vi "AttrMap-Merge.vi"(6 "If exist? Skip(T)/Overwrite(F)":bool=TRUE, 8 "error in (no error)":errorcluster, 10 "AttrMap B":T1, 11 "AttrMap A":T1) -> (0 "error out":errorcluster, 3 "AttrMap A after B->A":T1)   [LabVIEW 2019, in "lv-apt-json-file.lvlib"]
uses:
  lv-apt-json-file.lvlib
  Typedef/Def-AttrMap.ctl
  f16f814e-f0a0-47f4-ae2a-f78fd01390a2.vi
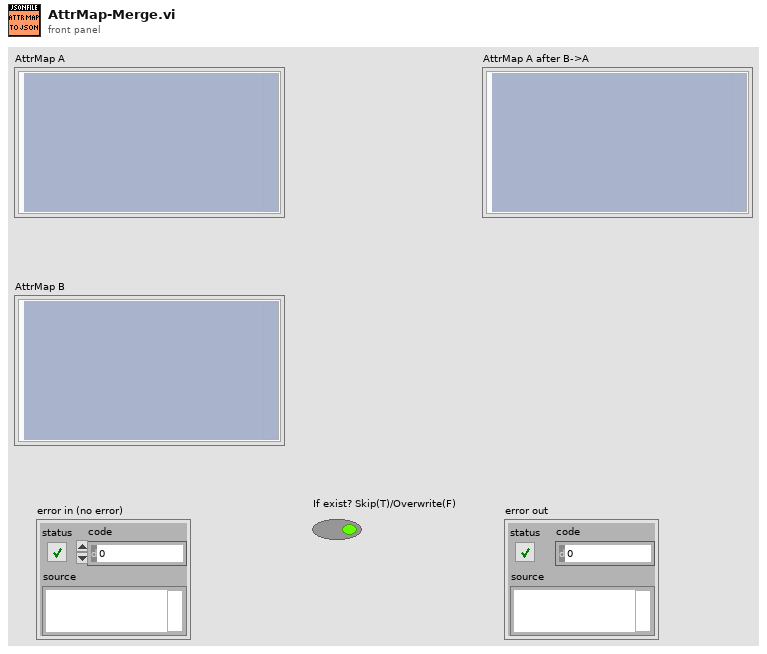
[diagram p1: front panel]
types:
  T1 = typedef "lv-apt-json-file.lvlib/Def-AttrMap.ctl" = cluster{"Map":variant}
  T2 = typedef "lv-apt-json-file.lvlib/Def-NameMap.ctl" = variant[]
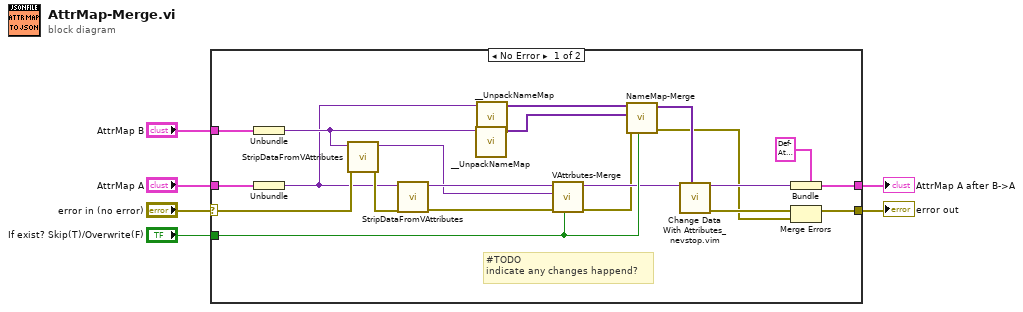
[diagram p0: block diagram]
diagram:
  n1 = case shown="No Error" "error in (no error)" {
    selector: "error in (no error)" -> [w11 w29]
    tunnel: "AttrMap A" -> [w27 w28]
    tunnel: "AttrMap B" -> [w26 _]
    tunnel: "If exist? Skip(T)/Overwrite(F)" -> [w21 _]
    tunnel: [w15 w29] -> w2
    tunnel: [w24 w28] -> w1
    frame No Error {
      # "#TODO \nindicate any changes happend?"
      n2 = Unbundle(w26) -> ("Map"=w9:variant)
      n3 = Unbundle(w27) -> ("Map"=w8:variant)
      n4 = call "StripDataFromVAttributes.vi"("error in (no error)"=w11, "Map"=w9) -> ("error out"=w10:errorcluster, "duplicate variant"=w7:variant)  [unwired: 8 in]
      n5 = call "StripDataFromVAttributes.vi"("error in (no error)"=w10, "Map"=w8) -> ("error out"=w12:errorcluster, "duplicate variant"=w13:variant)  [unwired: 8 in]
      n6 = call "__UnpackNameMap.vi"("Map"=w9) -> ("NameMap"=w17:T2)  [unwired: 10 in]
      n7 = call "__UnpackNameMap.vi"("Map"=w8) -> ("NameMap"=w18:T2)  [unwired: 10 in]
      n8 = call "VAttrbutes-Merge.vi"("If exist? Skip(T)/Overwrite(F)"=w21, "error in (no error)"=w12, "VAttributes B"=w7, "VAttributes A"=w13) -> ("error out"=w19:errorcluster, "VAttributes A after B->A"=w20:variant)  [unwired: 6 in]
      n9 = call "NameMap-Merge.vi"("If exist? Skip(T)/Overwrite(F)"=w21, "error in (no error)"=w19, "NameMap B"=w17, "NameMap A"=w18) -> ("error out"=w14:errorcluster, "NameMap A after B->A"=w22:T2)  [unwired: 6 in]
      n10 = call "Change Data With Attributes_nevstop.vim"("Data"=w22, "Variant in"=w20) -> ("error out"=w16:errorcluster, "Variant out"=w25:variant)  [unwired: 8 in]
      n11 = Bundle(cluster=T1 {"Map"=variant} ("AttrMap"), "Map"=w25) -> (w24:T1)
      n12 = Merge Errors(w16, w14) -> (w15:errorcluster)
    }
    frame Error {
    }
  }
  "AttrMap A after B->A" <- w1
  "error out" <- w2
